vi "Measurement_Type_selector_UI_String_to_enum.vi"(8 "error in (no error)":errorcluster, 11 "Measurement Type":string) -> (0 "error out":errorcluster, 3 "AvgMinMax":enum16{"Average", "Max", "Min", "Max2"}(ring))   [LabVIEW 2014]
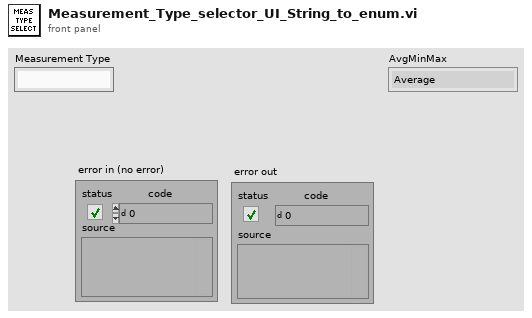
[diagram p1: front panel]
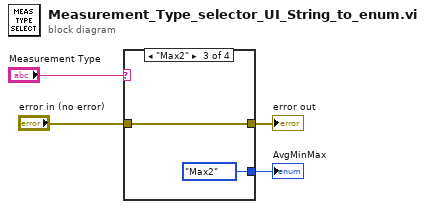
[diagram p0: block diagram]
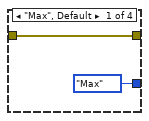
[diagram p2: hidden frame]
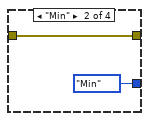
[diagram p3: hidden frame]
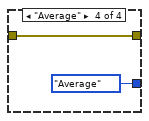
[diagram p4: hidden frame]
diagram:
  n1 = case shown="\"Max2\"" "Measurement Type" {
    tunnel: [enum16{"Average", "Max", "Min", "Max2"}."Max" ("AvgMinMax") enum16{"Average", "Max", "Min", "Max2"}."Min" ("AvgMinMax") enum16{"Average", "Max", "Min", "Max2"}."Max2" ("AvgMinMax") enum16{"Average", "Max", "Min", "Max2"}."Average" ("AvgMinMax")] -> w4
    tunnel: "error in (no error)" -> [w5 w7 w9 w11]
    tunnel: [w5 w7 w9 w11] -> w1
    frame "Max", Default {
    }
    frame "Min" {
    }
    frame "Max2" {
    }
    frame "Average" {
    }
  }
  "AvgMinMax" <- w4
  "error out" <- w1
